vi "Ctor.vi"(8 "error in (no error)":errorcluster, 11 "AudioMonPanel in":refnum<class "AudioMonPanel.lvclass">) -> (0 "error out":errorcluster, 3 "AudioMonPanel out":refnum<class "AudioMonPanel.lvclass">)   [LabVIEW 2022 SP3, in "TouchControl.lvlib" / "AudioMonPanel.lvclass"]
uses:
  AudioMonPanel.lvclass
  <vilib>/IlluminatedG/IG OOPanel/OOPanel/Panel/Panel.lvclass
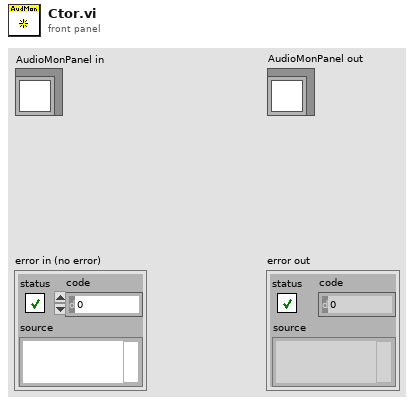
[diagram p1: front panel]
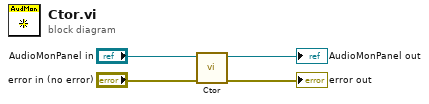
[diagram p0: block diagram]
diagram:
  n1 = call-parent "Ctor.vi"("error in (no error)"="error in (no error)", "Panel in"="AudioMonPanel in") -> ("error out"=→"error out":errorcluster, "Panel out"=→"AudioMonPanel out":refnum<class "AudioMonPanel.lvclass">)  [unwired: 8 in]
